vi "Main.vi"() -> ()   [LabVIEW 2021]
doc: "The myRIO Project template acquires acceleration data from the onboard accelerometer and displays the changes of acceleration values in a waveform chart."
uses:
  <vilib>/vision/driver/IMAQdx.llb/IMAQdx Camera Control Mode.ctl
  <vilib>/vision/driver/IMAQdx.llb/IMAQdx Acquisition Mode.ctl
  <vilib>/vision/driver/IMAQdx.llb/IMAQdx Buffer Number Mode.ctl
  <vilib>/userDefined/High Color/IMAQdx.ctl
  <vilib>/myRIO/Instrument Drivers/Onboard IO/PWM/typedefs/PWM Reference.ctl
  <vilib>/myRIO/Common/Instrument Driver Framework/Utilities/typedefs/myRIO Generic Hardware Reference.ctl
  <vilib>/myRIO/Common/Instrument Driver Framework/Utilities/typedefs/Hardware Version Enum.ctl
  <vilib>/myRIO/Common/Instrument Driver Framework/Utilities/typedefs/myRIO v1.0 Reference.ctl
  <vilib>/myRIO/Common/Instrument Driver Framework/Utilities/typedefs/Generic FPGA Reference.ctl
  <vilib>/myRIO/Common/Instrument Driver Framework/myRIO v1.0/PWM/typedefs/PWM Channels Enum.ctl
  <vilib>/myRIO/Instrument Drivers/Onboard IO/PWM/typedefs/PWM Configuration.ctl
  <vilib>/userDefined/High Color/nirio_resource_hc.ctl
  <vilib>/myRIO/Instrument Drivers/Onboard IO/DIO/typedefs/DIO Reference.ctl
  <vilib>/myRIO/Common/Instrument Driver Framework/myRIO v1.0/DIO/typedefs/DIO Channels List.ctl
  <vilib>/myRIO/Common/Instrument Driver Framework/myRIO v1.0/DIO/typedefs/DIO Channels Enum.ctl
  <vilib>/myRIO/Instrument Drivers/Onboard IO/AI/typedefs/AI Reference.ctl
  <vilib>/myRIO/Common/Instrument Driver Framework/myRIO v1.0/AI/typedefs/AI Channels List.ctl
  <vilib>/myRIO/Common/Instrument Driver Framework/myRIO v1.0/AI/typedefs/AI Channels Enum.ctl
  <vilib>/myRIO/Common/Instrument Driver Framework/Utilities/typedefs/Analog Scaling Constants List.ctl
  <vilib>/myRIO/Common/Instrument Driver Framework/Utilities/typedefs/Analog Scaling Constants.ctl
  <vilib>/myRIO/Common/Instrument Driver Framework/myRIO v1.0/PWM/vis/myRIO v1.1 Open PWM.vi
  <vilib>/myRIO/Common/Instrument Driver Framework/myRIO v1.0/DIO/vis/myRIO v1.1 Open DIO.vi
  <vilib>/myRIO/Common/Instrument Driver Framework/Utilities/vis/Is FPGA Ref Available.vi
  <vilib>/myRIO/Common/Instrument Driver Framework/myRIO v1.0/AI/vis/myRIO v1.1 Open AI.vi
  <vilib>/myRIO/Common/Instrument Driver Framework/Utilities/vis/Validate Channels.vi
  <vilib>/myRIO/Common/Instrument Driver Framework/myRIO v1.0/PWM/vis/myRIO v1.0 Reserve PWM.vi
  <vilib>/myRIO/Instrument Drivers/Onboard IO/PWM/vis/Set Duty Cycle and Frequency.vi
  <vilib>/myRIO/Common/Instrument Driver Framework/myRIO v1.0/DIO/vis/myRIO v1.0 Reserve DIO.vi
  <vilib>/myRIO/Common/Instrument Driver Framework/myRIO v1.0/AI/vis/myRIO v1.0 Reserve AI.vi
  <vilib>/myRIO/Common/Instrument Driver Framework/myRIO v1.0/PWM/vis/myRIO v1.0 Close PWM.vi
  <vilib>/myRIO/Common/Instrument Driver Framework/myRIO v1.0/DIO/vis/myRIO v1.0 Close DIO.vi
  <vilib>/myRIO/Common/Instrument Driver Framework/myRIO v1.0/AI/vis/myRIO v1.0 Close AI.vi
  <vilib>/myRIO/Common/Instrument Driver Framework/myRIO v1.0/PWM/vis/myRIO v1.0 Build MUX Configuration PWM.vi
  <vilib>/myRIO/Common/Instrument Driver Framework/myRIO v1.0/Resource Manager/vis/myRIO v1.0 Reserve Channel List.vi
  <vilib>/myRIO/Common/Instrument Driver Framework/myRIO v1.0/DIO/vis/myRIO v1.0 Build MUX Configuration DIO.vi
  <vilib>/myRIO/Common/Instrument Driver Framework/myRIO v1.0/AI/vis/myRIO v1.0 Build MUX Configuration AI.vi
  <vilib>/myRIO/Common/Instrument Driver Framework/myRIO v1.0/PWM/vis/myRIO v1.0 Unreserve PWM.vi
  <vilib>/myRIO/Common/Instrument Driver Framework/myRIO v1.0/DIO/vis/myRIO v1.0 Unreserve DIO.vi
  <vilib>/myRIO/Common/Instrument Driver Framework/myRIO v1.0/AI/vis/myRIO v1.0 Unreserve AI.vi
  <vilib>/myRIO/Common/Instrument Driver Framework/myRIO v1.0/Resource Manager/vis/myRIO v1.0 Create Configuration List.vi
  <vilib>/myRIO/Common/Instrument Driver Framework/myRIO v1.0/Resource Manager/vis/myRIO v1.0 Reserve Channel.vi
  <vilib>/myRIO/Common/Instrument Driver Framework/myRIO v1.0/Resource Manager/vis/myRIO v1.0 Unreserve Channel.vi
  <vilib>/myRIO/Common/Instrument Driver Framework/myRIO v1.0/Resource Manager/vis/myRIO v1.0 Unreserve Channel List.vi
  <vilib>/myRIO/Common/Instrument Driver Framework/myRIO v1.0/Resource Manager/vis/myRIO v1.0 Build Mutex Name.vi
  <vilib>/Utility/VariantDataType/GetNumericInfo.vi
  <vilib>/Utility/error.llb/Error Cluster From Error Code.vi
  <vilib>/myRIO/Common/Instrument Driver Framework/myRIO v1.0/myRIO v1.1 Open.vi
  <vilib>/myRIO/Common/Instrument Driver Framework/Utilities/vis/IO Manager.vi
  <vilib>/myRIO/Common/Instrument Driver Framework/Utilities/vis/Configuration Manager.vi
  <vilib>/myRIO/Common/Instrument Driver Framework/myRIO v1.0/Resource Manager/vis/myRIO v1.0 Configure IO.vi
  <vilib>/myRIO/Common/Instrument Driver Framework/myRIO v1.0/myRIO v1.0 Close.vi
  <vilib>/myRIO/Common/Instrument Driver Framework/myRIO v1.0/DIO/vis/myRIO v1.0 Read DIO.vi
  <vilib>/myRIO/Common/Instrument Driver Framework/myRIO v1.0/PWM/vis/myRIO v1.0 Write PWM.vi
  <vilib>/myRIO/Common/Instrument Driver Framework/myRIO v1.0/AI/vis/myRIO v1.0 Get Scaling Constants AI.vi
  <vilib>/myRIO/Common/Instrument Driver Framework/myRIO v1.0/AI/vis/myRIO v1.0 Read AI.vi
  <vilib>/myRIO/Common/Instrument Driver Framework/myRIO v1.0/DIO/vis/myRIO v1.0 Write DIO.vi
  <vilib>/myRIO/Common/Instrument Driver Framework/myRIO v1.0/PWM/vis/myRIO v1.0 Shutdown PWM.vi
  <vilib>/myRIO/Common/Instrument Driver Framework/myRIO v1.0/DIO/vis/myRIO v1.0 Shutdown DIO.vi
  <vilib>/myRIO/Express VI/Onboard Devices/Button/Button Express VI.xnode
  <vilib>/myRIO/Instrument Drivers/Onboard IO/DIO/vis/myRIO DIO Open.xnode
  <vilib>/myRIO/Instrument Drivers/Onboard IO/PWM/vis/myRIO PWM Open.xnode
  <vilib>/myRIO/Instrument Drivers/Onboard IO/AI/vis/myRIO AI Open.xnode
  <vilib>/myRIO/Express VI/Onboard Devices/LED/LED Express VI.xnode
  <vilib>/vision/driver/NI_Vision_Acquisition_Software.lvlib
  <vilib>/vision/NI_Vision_Development_Module.lvlib
  <vilib>/myRIO/Instrument Drivers/Onboard IO/PWM/PWM.lvlib
  <vilib>/myRIO/Instrument Drivers/Onboard IO/AI/AI.lvlib
  <vilib>/myRIO/Instrument Drivers/Onboard IO/DIO/DIO.lvlib
panel:
  in  "error in 3":errorcluster
  in  "?":errorcluster
  in  "port":dbl
  in  "IP":string
  in  "error in (no error)":errorcluster
  out "Numeric":dbl
  out "String":string
  in  "Boolean":bool
  in  "error in 2":errorcluster
  out "darkness scale":dbl(slide) scale=0.0..10.0
  in  "ROI Descriptor":T1 {"Contours"."Type" items=["No Selection", "Point", "Line", "Rectangle", "Oval", "Polygon", "Freehand Region", "Annulus", "Unused2", "Unused3", "Broken Line", "Freehand Line", "Rotated Rectangle"]}
  in  "error in":errorcluster
  in  "stop":bool
  out "Colour Value":u32
  out "Color Box":u32(colorbox)
  out "Image 2":T2(plugin-control)
  out "circles":i32
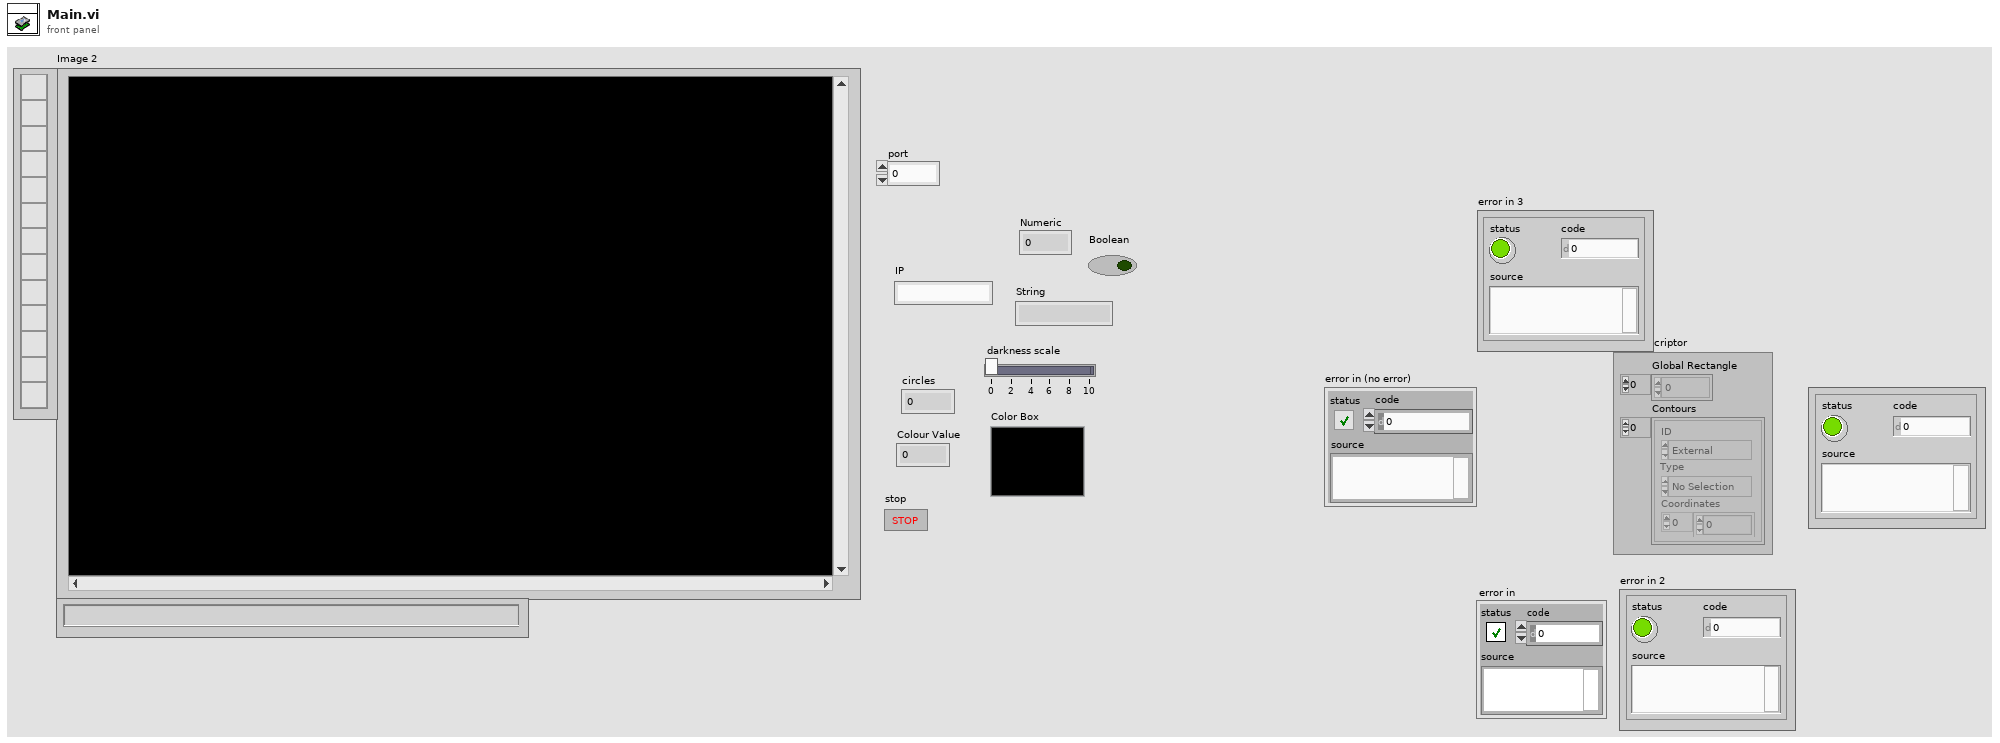
[diagram p1: front panel]
types:
  T1 = cluster{"Global Rectangle":i32[], "Contours":cluster{"ID":enum32{"External", "Internal"}, "Type":u32, "Coordinates":i32[]}[]}
  T2 = typedef "IMAQ Image.ctl" = refnum<image>
  T3 = typedef "IMAQ Rectangle" = cluster{"Left":i32, "Top":i32, "Right":i32, "Bottom":i32, "Rotation":dbl}
  T4 = typedef "IMAQdx.ctl" = refnum<k21>
  T5 = typedef "NI_Vision_Acquisition_Software.lvlib/IMAQdx Buffer Number Mode.ctl" = enum32{"Next", "Last", "Buffer Number", "Every", "Last New"}
  T6 = typedef "NI_Vision_Acquisition_Software.lvlib/IMAQdx Acquisition Mode.ctl" = enum32{"One Shot", "Continuous"}
  T7 = typedef "NI_Vision_Acquisition_Software.lvlib/IMAQdx Camera Control Mode.ctl" = enum32{"Controller", "Listener"}
  T8 = typedef "AI.lvlib/AI Reference.ctl" = cluster{"myRIO Reference":T9, "AI Channels List":T13, "AI Scaling Constants List":T15}
  T9 = typedef "myRIO Generic Hardware Reference.ctl" = cluster{"myRIO Model":T10, "myRIO Hardware Reference":T11}
  T10 = typedef "Hardware Version Enum.ctl" = enum16{"Unknown", "myRIO-1900", "myRIO-1950", "roboRIO", "NI ELVIS RIO CM", "ELVIS III"}
  T11 = typedef "myRIO v1.0 Reference.ctl" = cluster{"Generic FPGA Reference":T12, "Allow multiple opens":bool}
  T12 = typedef "Generic FPGA Reference.ctl" = refnum<k20>
  T13 = typedef "AI Channels List.ctl" = T14[]
  T14 = typedef "AI Channels Enum.ctl" = enum16{"Not Connected", "AudioIn/Left", "AudioIn/Right", "C/AI0", "C/AI1", "A/AI0", "A/AI1", "A/AI2", "A/AI3", "A/AI4", "A/AI5", "A/AI6", "A/AI7", "B/AI0", "B/AI1", "B/AI2", "B/AI3", "B/AI4", "B/AI5", "B/AI6", "B/AI7", "AI/AI0", "AI/AI1", "AI/AI2", "AI/AI3", "A/AI0 (DIFF)", "A/AI1 (DIFF)", "A/AI2 (DIFF)", "A/AI3 (DIFF)", "B/AI0 (DIFF)", "B/AI1 (DIFF)", "B/AI2 (DIFF)", "B/AI3 (DIFF)"}
  T15 = typedef "Analog Scaling Constants List.ctl" = T16[]
  T16 = typedef "Analog Scaling Constants.ctl" = cluster{"LSB Weight (Volts)":dbl, "Offset (Volts)":dbl, "Signed?":bool}
  T17 = typedef "PWM.lvlib/PWM Reference.ctl" = cluster{"myRIO Reference":T9, "PWM Channels Enum":T18, "PWM Configuration":T19}
  T18 = typedef "PWM Channels Enum.ctl" = enum16{"Not Connected", "C/PWM0", "C/PWM1", "A/PWM0", "A/PWM1", "A/PWM2", "A/PWM3", "A/PWM4", "A/PWM5", "A/PWM6", "A/PWM7", "A/PWM8", "A/PWM9", "A/PWM10", "A/PWM11", "A/PWM12", "A/PWM13", "A/PWM14", "A/PWM15", "A/PWM16", "A/PWM17", "A/PWM18", "A/PWM19", "B/PWM0", "B/PWM1", "B/PWM2", "B/PWM3", "B/PWM4", "B/PWM5", "B/PWM6", "B/PWM7", "B/PWM8", "B/PWM9", "B/PWM10", "B/PWM11", "B/PWM12", "B/PWM13", "B/PWM14", "B/PWM15", "B/PWM16", "B/PWM17", "B/PWM18", "B/PWM19", "PWM/PWM0", "PWM/PWM1", "PWM/PWM2", "PWM/PWM3", "PWM/PWM4", "PWM/PWM5", "PWM/PWM6", "PWM/PWM7", "PWM/PWM8", "PWM/PWM9"}
  T19 = typedef "PWM.lvlib/PWM Configuration.ctl" = cluster{"Frequency":dbl, "Duty Cycle":dbl}
  T20 = typedef "DIO.lvlib/DIO Reference.ctl" = cluster{"myRIO Reference":T9, "DIO Channels List":T21}
  T21 = typedef "DIO Channels List.ctl" = T22[]
  T22 = typedef "DIO Channels Enum.ctl" = enum16{"Not Connected", "C/DIO0", "C/DIO1", "C/DIO2", "C/DIO3", "C/DIO4", "C/DIO5", "C/DIO6", "C/DIO7", "A/DIO0", "A/DIO1", "A/DIO2", "A/DIO3", "A/DIO4", "A/DIO5", "A/DIO6", "A/DIO7", "A/DIO8", "A/DIO9", "A/DIO10", "A/DIO11", "A/DIO12", "A/DIO13", "A/DIO14", "A/DIO15", "A/DIO16", "A/DIO17", "A/DIO18", "A/DIO19", "B/DIO0", "B/DIO1", "B/DIO2", "B/DIO3", "B/DIO4", "B/DIO5", "B/DIO6", "B/DIO7", "B/DIO8", "B/DIO9", "B/DIO10", "B/DIO11", "B/DIO12", "B/DIO13", "B/DIO14", "B/DIO15", "B/DIO16", "B/DIO17", "B/DIO18", "B/DIO19", "LED0", "LED1", "LED2", "LED3", "Button0", "DIO/DIO0", "DIO/DIO1", "DIO/DIO2", "DIO/DIO3", "DIO/DIO4", "DIO/DIO5", "DIO/DIO6", "DIO/DIO7", "DIO/DIO8", "DIO/DIO9", "SPI/CS0", "SPI/CS1", "SPI/CS2", "SPI/CS3", "LED RADIO (Green)", "LED RADIO (Red)", "LED COMM (Green)", "LED COMM (Red)", "LED MODE (Green)", "LED MODE (Red)"}
  T23 = typedef "nirio_resource_hc.ctl" = tag
  T24 = typedef "Image Type" = u32
  T25 = typedef "ROI Descriptor" = cluster{"Global Rectangle":i32[], "Contours":cluster{"ID":enum32{"External", "Internal"}, "Type":u32, "Coordinates":i32[]}[]}
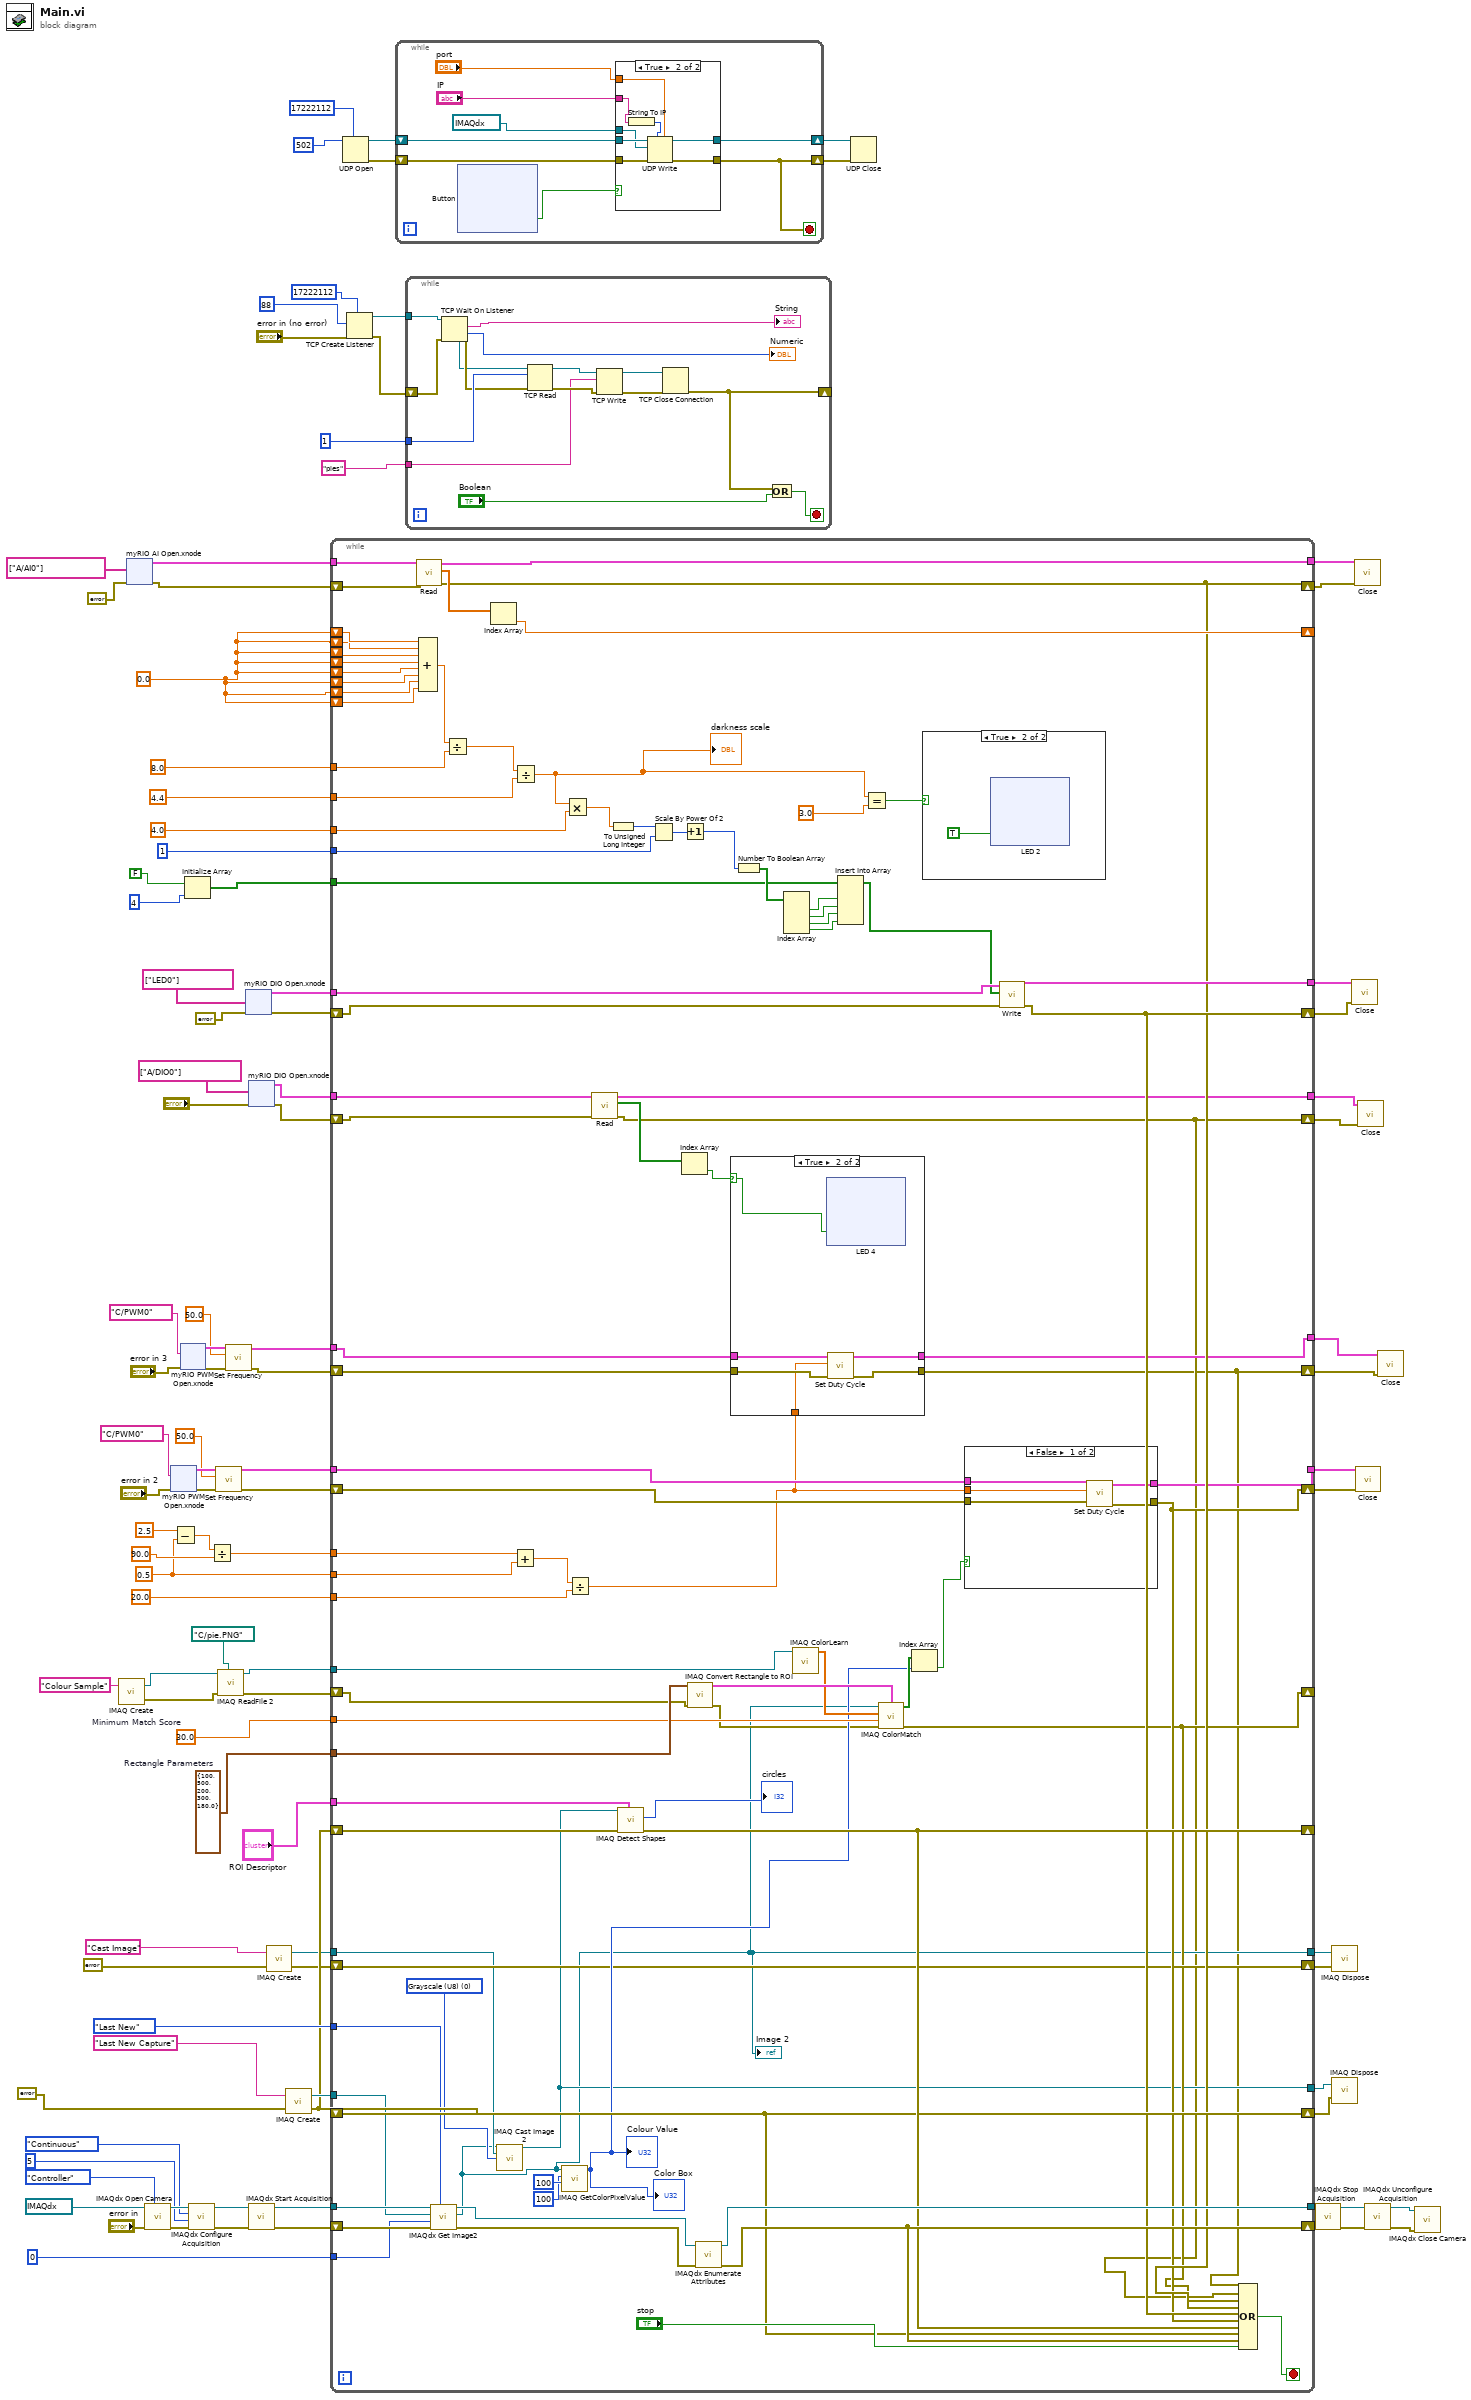
[diagram p0: block diagram]
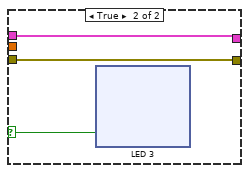
[diagram p4: hidden frame]
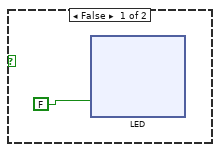
[diagram p5: hidden frame]
diagram:
  w25 = 30.0  # Minimum Match Score
  w26 = T3 {"Left"=100, "Top"=500, "Right"=200, "Bottom"=300, "Rotation"=180.0}  # Rectangle Parameters
  w57 = 0.5
  w43 = 0.0
  n1 = call "IMAQ Create"("Image Name"="Colour Sample") -> ("New Image"=w29:T2, "error out"=w28:errorcluster)  [unwired: 4 in]
  n2 = xnode "myRIO AI Open.xnode"("error in (no error)"=errorcluster {"status"=FALSE, "code"=0, "source"=""}, "Channel Names"=tag[] ["A/AI0"]) -> ("error out"=w45:errorcluster, "AI Ref Out"=w47:T8)  [unwired: 1 in]
  n3 = call <vilib>:"IMAQdx Open Camera.vi"("Camera Control Mode"=IMAQdx_Camera_Control_Mode."Controller", "error in"="error in", "Session In"=T4 "cam1") -> ("error out"=w96:errorcluster, "Session Out"=w97:T4)  [unwired: 7 in]
  n4 = xnode "myRIO PWM Open.xnode"("error in (no error)"="error in 2", "Channel Name"=tag "C/PWM0") -> ("error out"=w76:errorcluster, "PWM Ref Out"=w75:T17)  [unwired: 1 in]
  n5 = Subtract(x=2.5, y=w57) -> (x-y=w72:dbl)
  n6 = xnode "myRIO PWM Open.xnode"("error in (no error)"="error in 3", "Channel Name"=tag "C/PWM0") -> ("error out"=w9:errorcluster, "PWM Ref Out"=w8:T17)  [unwired: 1 in]
  n7 = Initialize Array(FALSE, 4) -> (w52:bool[])
  n8 = call <vilib>:"IMAQdx Configure Acquisition.vi"("error in"=w96, "Number of Buffers"=u32 5, "Continuous?"=IMAQdx_Acquisition_Mode."Continuous", "Session In"=w97) -> ("error out"=w103:errorcluster, "Session Out"=w102:T4)  [unwired: 6 in]
  n9 = Divide(x=w72, y=90.0) -> (x/y=w63:dbl)
  n10 = call <vilib>:"Set Frequency.vi"("error in (no error)"=w76, "Frequency [Hz]"=50.0, "PWM Ref In"=w75) -> ("error out"=w62:errorcluster, "PWM Ref Out"=w61:T17)  [unwired: 6 in]
  n11 = call "IMAQ ReadFile 2"("File Path"=path "C:/pie.PNG", "error in (no error)"=w28, "Image"=w29) -> ("error out"=w18:errorcluster, "Image Out"=w27:T2)  [unwired: 4 in, 3 out]
  n12 = call <vilib>:"Set Frequency.vi"("error in (no error)"=w9, "Frequency [Hz]"=50.0, "PWM Ref In"=w8) -> ("error out"=w4:errorcluster, "PWM Ref Out"=w3:T17)  [unwired: 6 in]
  n13 = xnode "myRIO DIO Open.xnode"("error in (no error)"=errorcluster {"status"=FALSE, "code"=0, "source"=""}, "Channel Names"=tag[] ["LED0"]) -> ("error out"=w56:errorcluster, "DIO Ref Out"=w55:T20)  [unwired: 1 in]
  n14 = xnode "myRIO DIO Open.xnode"("error in (no error)"="?", "Channel Names"=tag[] ["A/DIO0"]) -> ("error out"=w14:errorcluster, "DIO Ref Out"=w15:T20)  [unwired: 1 in]
  n15 = call <vilib>:"IMAQdx Start Acquisition.vi"("error in"=w103, "Session In"=w102) -> ("error out"=w90:errorcluster, "Session Out"=w91:T4)  [unwired: 8 in]
  n16 = call "IMAQ Create"("Image Name"="Cast Image", "error in (no error)"=errorcluster {"status"=FALSE, "code"=0, "source"=""} ("error in")) -> ("New Image"=w21:T2, "error out"=w23:errorcluster)  [unwired: 3 in]
  n17 = call "IMAQ Create"("Image Name"="Last New Capture", "error in (no error)"=errorcluster {"status"=FALSE, "code"=0, "source"=""} ("error in")) -> ("New Image"=w87:T2, "error out"=w78:errorcluster)  [unwired: 3 in]
  n18 = while {
    tunnel: w91 -> [w194]
    shift-right: [w179] -> w85
    shift-left: w90 -> [w193]
    tunnel: w87 -> [w192]
    shift-right: [w177] -> w86
    shift-left: w78 -> [w177]
    tunnel: [w116] -> w84
    tunnel: [w191] -> w83
    tunnel: u32 0 ("Buffer Number In") -> [w189]
    shift-right: [w178] -> _
    shift-left: w78 -> [w183]
    tunnel: IMAQdx_Buffer_Number_Mode."Last New" ("Buffer Number Mode (Next)") -> [w188]
    tunnel: "ROI Descriptor" -> [w182]
    tunnel: w63 -> [w163]
    shift-right: [w125] -> w60
    shift-left: w62 -> [w127]
    tunnel: w61 -> [w128]
    tunnel: [w126] -> w59
    tunnel: 20.0 -> [w161]
    tunnel: w57 -> [w160]
    shift-right: [w138] -> w54
    shift-left: w56 -> [w158]
    tunnel: w55 -> [w159]
    tunnel: [w157] -> w53
    tunnel: w52 -> [w156]
    tunnel: 8.0 -> [w155]
    tunnel: 4.4 -> [w154]
    tunnel: 4.0 -> [w153]
    tunnel: 1 -> [w152]
    tunnel: w47 -> [w151]
    tunnel: [w150] -> w46
    shift-right: [w137] -> w44
    shift-left: w45 -> [w149]
    shift-right: [w141] -> _
    shift-left: w43 -> [w148]
    shift-left: w43 -> [w135]
    shift-left: w43 -> [w134]
    shift-left: w43 -> [w147]
    shift-left: w43 -> [w146]
    shift-left: w43 -> [w145]
    shift-left: w43 -> [w144]
    shift-left: w43 -> [w143]
    tunnel: w27 -> [w131]
    tunnel: w26 -> [w133]
    tunnel: w25 -> [w132]
    shift-right: [w121] -> w20
    shift-left: w23 -> [w121]
    tunnel: w21 -> [w117]
    tunnel: [w115] -> w19
    shift-right: [w118] -> _
    shift-left: w18 -> [w120]
    tunnel: [w114] -> w16
    tunnel: w15 -> [w113]
    shift-right: [w105] -> w13
    shift-left: w14 -> [w112]
    shift-right: [w104] -> w5
    shift-left: w4 -> [w108]
    tunnel: w3 -> [w109]
    tunnel: [w107] -> w2
    stop <- w139 stop-if-true
    w184 = T24 0 items=["Grayscale (U8)", "Grayscale (I16)", "Grayscale (SGL)", "Complex (CSG)", "RGB (U32)", "HSL (U32)", "RGB (U64)", "Grayscale (U16)"] ("Image Type")
    n19 = call <vilib>:"Read.vi"("error in (no error)"=w149, "AI Ref In"=w151) -> ("error out"=w137:errorcluster, "Values"=w142:dbl[], "AI Ref Out"=w150:T8)  [unwired: 7 in]
    n20 = Compound Arithmetic op=ADD(w148, w135, w134, w147, w146, w145, w144, w143) -> (w136:dbl)
    n21 = call <vilib>:"IMAQdx Get Image2.vi"("Buffer Number Mode (Next)"=w188, "error in"=w193, "Buffer Number In"=w189, "Image In"=w192, "Session In"=w194) -> ("error out"=w190:errorcluster, "Image Out"=w115:T2, "Session Out"=w185:T4)  [unwired: 3 in, 1 out]
    "Image 2" <- w115
    n22 = Divide(x=w136, y=w155) -> (x/y=w165:dbl)
    n23 = Index Array(array=w142) -> (element=w141:dbl)  [unwired: 1 in]
    n24 = call "IMAQ Cast Image 2"("Image Src"=w115, "Image Dst"=w117, "Image Type"=w184) -> ("Image Dst Out"=w116:T2)  [unwired: 11 in, 1 out]
    n25 = Add(x=w163, y=w160) -> (x+y=w162:dbl)
    n26 = Divide(x=w165, y=w154) -> (x/y=w176:dbl)
    "darkness scale" <- w176
    n27 = call "IMAQ GetColorPixelValue"("Y Coordinate"=100, "X Coordinate"=100, "Image"=w115) -> ("Pixel Value (U32)"=w122:u32)  [unwired: 1 in, 2 out]
    "Colour Value" <- w122
    "Color Box" <- w122
    n28 = Multiply(x=w176, y=w153) -> (x*y=w166:dbl)
    n29 = Divide(x=w162, y=w161) -> (x/y=w106:dbl)
    n30 = call <vilib>:"Read.vi"("error in (no error)"=w112, "DIO Ref In"=w113) -> ("error out"=w105:errorcluster, "Values"=w111:bool[], "DIO Ref Out"=w114:T20)  [unwired: 7 in]
    n31 = To Unsigned Long Integer(number=w166) -> (unsigned 32bit integer=w167:u32)
    n32 = call-poly "IMAQ Detect Shapes"("ROI Descriptor"=w182, "error in (no error)"=w183, "Image"=w116) -> ("error out"=w178:errorcluster, "Number of Matches Returned"=→"circles":i32)  [unwired: 6 in, 1 out]
    n33 = Scale By Power Of 2(n=w167, x=w152) -> (x*2^n=w168:i32)
    n34 = Index Array(array=w111) -> (element=w110:bool)  [unwired: 1 in]
    n35 = Increment(x=w168) -> (x+1=w169:i32)
    n36 = call "IMAQ Convert Rectangle to ROI"("error in (no error)"=w120, "Rectangle"=w133) -> ("error out"=w119:errorcluster, "ROI Descriptor"=w130:T25)  [unwired: 7 in]
    n37 = call <vilib>:"IMAQdx Enumerate Attributes.vi"("error in"=w190, "Session In"=w185) -> ("error out"=w179:errorcluster, "Session Out"=w191:T4)  [unwired: 7 in, 1 out]
    n38 = case shown="True" w110 {
      selector: w110 -> [_ w202]
      tunnel: w109 -> [w196 w201]
      tunnel: w108 -> [w195 w200]
      tunnel: [w196 w199] -> w107
      tunnel: [w195 w198] -> w104
      tunnel: w106 -> [_ w197]
      frame False {
      }
      frame True {
        n39 = xnode "LED 4"("LED2"=w202) -> ()  [unwired: 1 in, 1 out]
        n40 = call <vilib>:"Set Duty Cycle.vi"("error in (no error)"=w200, "Duty Cycle"=w197, "PWM Ref In"=w201) -> ("error out"=w198:errorcluster, "PWM Ref Out"=w199:T17)  [unwired: 6 in]
      }
    }
    n41 = Number To Boolean Array(number=w169) -> (Boolean array=w170:bool[])
    n42 = Index Array(array=w170) -> (element #1=w171:bool, element #2=w172:bool, element #3=w173:bool, element #4=w174:bool)  [unwired: 4 in]
    n43 = call "IMAQ ColorLearn"("Image"=w131) -> ("Color Spectrum"=w129:dbl[])  [unwired: 7 in, 1 out]
    n44 = Insert Into Array(array=w156, new element #1=w171, new element #2=w172, new element #3=w173, new element #4=w174) -> (w140:bool[])  [unwired: 1 in]
    n45 = Equal?(x=w176, y=3.0) -> (x = y?=w175:bool)
    n46 = call "IMAQ ColorMatch"("ROI Descriptor"=w130, "Image"=w115, "Color Spectrum"=w129, "Minimum Match Score"=w132, "error in (no error)"=w119) -> ("Match Flag"=w124:bool[], "error out"=w118:errorcluster)  [unwired: 2 in, 1 out]
    n47 = Index Array(array=w124, index=w122) -> (element=w123:bool)
    n48 = case shown="True" w175 {
      frame False {
        n49 = xnode "LED"("LED0"=FALSE) -> ()  [unwired: 1 in, 1 out]
      }
      frame True {
        n50 = xnode "LED 2"("LED0"=TRUE) -> ()  [unwired: 1 in, 1 out]
      }
    }
    n51 = case shown="False" w123 {
      selector: w123 -> [_ w243]
      tunnel: w128 -> [w241 w245]
      tunnel: w127 -> [w242 w244]
      tunnel: [w240 w245] -> w126
      tunnel: [w239 w244] -> w125
      tunnel: w106 -> [w238 _]
      frame False {
        n52 = call <vilib>:"Set Duty Cycle.vi"("error in (no error)"=w242, "Duty Cycle"=w238, "PWM Ref In"=w241) -> ("error out"=w239:errorcluster, "PWM Ref Out"=w240:T17)  [unwired: 6 in]
      }
      frame True {
        n53 = xnode "LED 3"("LED3"=w243) -> ()  [unwired: 1 in, 1 out]
      }
    }
    n54 = call <vilib>:"Write.vi"("error in (no error)"=w158, "Values"=w140, "DIO Ref In"=w159) -> ("error out"=w138:errorcluster, "DIO Ref Out"=w157:T20)  [unwired: 6 in]
    n55 = Compound Arithmetic op=OR(w104, w105, w118, w137, w138, w125, w178, w177, w179, "stop") -> (w139:bool)
  }
  n56 = UDP Open(7:17222112, 11:502) -> (port=w36:refnum<k16>, 0:w35:errorcluster)  [unwired: 3 in, 1 out]
  n57 = TCP Create Listener(7:17222112, 8:"error in (no error)", 10:88) -> (0:w37:errorcluster, 3:w38:refnum<k5>)  [unwired: 2 in, 1 out]
  n58 = while {
    shift-right: [w357] -> w34
    shift-left: w35 -> [w359]
    shift-right: [w358] -> w32
    shift-left: w36 -> [w360]
    stop <- w357 stop-if-true
    n59 = xnode "Button"() -> ("Value"=w354:bool)  [unwired: 1 in, 1 out]
    n60 = case shown="True" w354 {
      tunnel: w360 -> [w397 w405]
      tunnel: [w397 w404] -> w358
      tunnel: w359 -> [w396 w403]
      tunnel: [w396 w402] -> w357
      tunnel: "port" -> [_ w401]
      tunnel: "IP" -> [_ w399]
      tunnel: T4 "cam1" ("Session In") -> [_ w398]
      frame False {
      }
      frame True {
        n61 = String To IP(1:w399) -> (0:w400:u32)
        n62 = UDP Write(address=w400, port or service name=w401, connection ID=w405, data in=w398, 8:w403) -> (error out=w402:errorcluster, 3:w404:refnum<k16>)  [unwired: 1 in]
      }
    }
  }
  n63 = while {
    shift-right: [w407] -> _
    shift-left: w37 -> [w408]
    tunnel: 1 -> [w420]
    tunnel: "pies" -> [w409]
    tunnel: w38 -> [w415]
    stop <- w410 stop-if-true
    n64 = TCP Wait On Listener(8:w408, 11:w415) -> (0:w414:errorcluster, 1:→"Numeric":u16, 2:→"String":string, 4:w406:refnum<k5>)  [unwired: 2 in, 1 out]
    n65 = TCP Read(connection ID=w406, bytes to read=w420, error in (no error)=w414) -> (connection ID out=w419:refnum<k5>, error out=w417:errorcluster)  [unwired: 2 in, 1 out]
    n66 = TCP Write(connection ID=w419, data in=w409, error in (no error)=w417) -> (connection ID out=w418:refnum<k5>, error out=w416:errorcluster)  [unwired: 1 in, 1 out]
    n67 = TCP Close Connection(connection ID=w418, error in (no error)=w416) -> (error out=w407:errorcluster)  [unwired: 1 in, 1 out]
    n68 = Compound Arithmetic op=OR(w407, "Boolean") -> (w410:bool)
  }
  n69 = UDP Close(connection ID=w32, 8:w34) -> ()  [unwired: 2 out]
  n70 = call <vilib>:"IMAQdx Stop Acquisition.vi"("error in"=w85, "Session In"=w83) -> ("error out"=w99:errorcluster, "Session Out"=w100:T4)  [unwired: 8 in]
  n71 = call "IMAQ Dispose"("Image"=w19, "error in (no error)"=w20) -> ()  [unwired: 4 in, 1 out]
  n72 = call "IMAQ Dispose"("Image"=w84, "error in (no error)"=w86) -> ()  [unwired: 4 in, 1 out]
  n73 = call <vilib>:"Close.vi"("error in (no error)"=w54, "DIO Ref In"=w53) -> ()  [unwired: 9 in, 1 out]
  n74 = call <vilib>:"Close.vi"("error in (no error)"=w44, "AI Ref In"=w46) -> ()  [unwired: 9 in, 1 out]
  n75 = call <vilib>:"Close.vi"("error in (no error)"=w60, "PWM Ref In"=w59) -> ()  [unwired: 9 in, 1 out]
  n76 = call <vilib>:"Close.vi"("error in (no error)"=w13, "DIO Ref In"=w16) -> ()  [unwired: 9 in, 1 out]
  n77 = call <vilib>:"IMAQdx Unconfigure Acquisition.vi"("error in"=w99, "Session In"=w100) -> ("error out"=w98:errorcluster, "Session Out"=w101:T4)  [unwired: 8 in]
  n78 = call <vilib>:"Close.vi"("error in (no error)"=w5, "PWM Ref In"=w2) -> ()  [unwired: 9 in, 1 out]
  n79 = call <vilib>:"IMAQdx Close Camera.vi"("error in"=w98, "Session In"=w101) -> ()  [unwired: 9 in, 1 out]
